vi "ContiAcq.vi"(4 "error in (no error)":errorcluster, 7 "Array":T1[](array[typedef])=[enum."S11", enum."S12", enum."S21", enum."S22"]) -> (0 "error out":errorcluster, 1 "Time":timestamp, 3 "SData":dbl[][](array[numeric]))   [LabVIEW 2023]
uses:
  LibreVNA/Types/Trace Enum.ctl
  LibreVNA/LibreVNA.lvclass
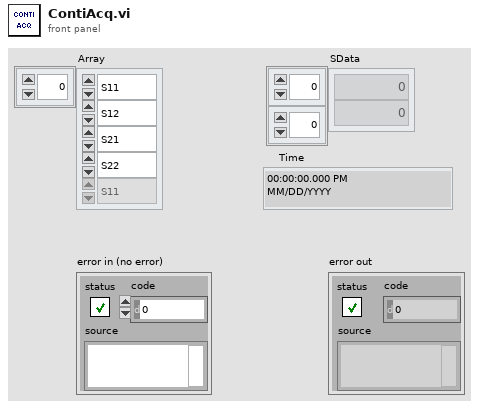
[diagram p1: front panel]
types:
  T1 = typedef "LibreVNA.lvclass/Trace Enum.ctl" = enum16{"S11", "S12", "S21", "S22"}
  T2 = typedef "UI Data.ctl" = cluster{"session":refnum<class "Modbus Master.lvclass">, "IsOpen":bool, "Timeout (ms)":i32, "TempFile":path, "LogStartTime":timestamp, "LibreVNA":refnum<class "LibreVNA.lvclass">, "VNAOpen":bool, "TempSP":dbl, "ActualTemp":dbl, "FileSaved":bool, "PIDOutput":dbl, "VNALogOpt":refnum<vi>, "PartName":string, "ComPort":refnum<visa-resource-name>, "S-Param Data":dbl[][], "VNADataFile - MAT":path, "VNADataFile - TDMS":path}
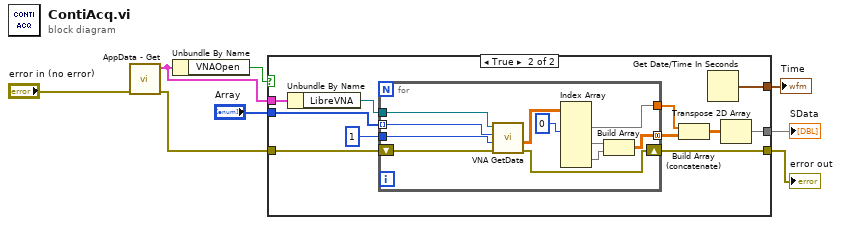
[diagram p0: block diagram]
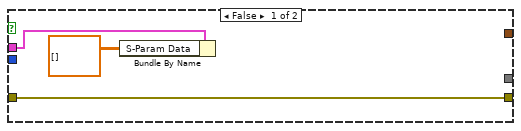
[diagram p2: hidden frame]
diagram:
  n1 = call "AppData - Get.vi"("error in"="error in (no error)") -> ("error out"=w3:errorcluster, "Data Out"=w5:T2)  [unwired: 5 in]
  n2 = Unbundle By Name(w5) -> ("VNAOpen"=w7:bool)
  n3 = case shown="True" w7 {
    tunnel: w3 -> [w11 w18]
    tunnel: [w11 w19] -> w8
    tunnel: "Array" -> [_ w22]
    tunnel: w5 -> [w10 w17]
    tunnel: [_ w13] -> w2
    tunnel: [_ w12] -> w1
    frame False {
      n4 = Bundle By Name(cluster=w10, "S-Param Data"=dbl[][] []) -> ()  [unwired: 1 out]
    }
    frame True {
      n5 = Unbundle By Name(w17) -> ("LibreVNA"=w16:refnum<class "LibreVNA.lvclass">)
      n6 = for {
        shift-right: [w31] -> w19
        shift-left: w18 -> [w32]
        tunnel: w22 -> [w30] mode=indexing
        tunnel: [w27] -> w21
        tunnel: [w25] -> w20 mode=concatenating
        tunnel: u32 1 ("command delay (ms)") -> [w23]
        tunnel: w16 -> [w33]
        n7 = call-dynamic "VNA GetData.vi"("error in (no error)"=w32, "command delay (ms)"=w23, "Trace Name"=w30, "LibreVNA in"=w33) -> ("error out"=w31:errorcluster, "Data Out"=w29:dbl[][])  [unwired: 2 in, 4 out]
        n8 = Index Array(array=w29, index (col) #1=0 ("disabled index (col)")) -> (element #1=w27:dbl[], element #2=w26:dbl[], element #3=w24:dbl[])  [unwired: 5 in]
        n9 = Build Array(w26, w24) -> (w25:dbl[][])
      }
      n10 = Build Array (concatenate)(w21, w20) -> (w14:dbl[][])
      n11 = Get Date/Time In Seconds() -> (seconds since 1Jan1904=w12:timestamp)
      n12 = Transpose 2D Array(2D array=w14) -> (transposed array=w13:dbl[][])
    }
  }
  "error out" <- w8
  "SData" <- w2
  "Time" <- w1
